vi "Initialize Single Node Browser.vi"(6 "Use Channel?":bool, 8 "error in (no error)":errorcluster, 9 "NodeName":string, 10 "Browser Ref 2":refnum<k24>, 11 "Item Ref in":T2 format="%.0x") -> (0 "error out":errorcluster, 2 "Browser Ref":T1, 3 "Item Ref out":T2 format="%.0x")   [LabVIEW 2015, in "Protection and Rolling Counter Addon System Explorer.lvlib"]
uses:
  <vilib>/NI Veristand/Custom Device API/Custom Device Item Ref.ctl
  NationalInstruments.VeriStand.SystemStorageUI
  <vilib>/NI Veristand/UI Controls/Single Node Browser/Single Node Browser Ref.ctl
  NationalInstruments.VeriStand.SystemStorage
  <vilib>/NI Veristand/Custom Device API/Get Item Property (Dependent Node Pointer).vi
  Protection and Rolling Counter Addon System Explorer.lvlib
  <vilib>/NI VeriStand/Custom Device Tools/Custom Device Utility Library/Custom Device Utility Library.lvlib
  <vilib>/NI VeriStand/Custom Device API/Custom Device API.lvlib
  <vilib>/NI Veristand/UI Controls/Single Node Browser/NI_VS UI Single Node Browser.lvlib
panel:
  in  "DisplayFilter":u8(ring)=7 items=["K_CHAN_R", "K_CHAN_W", "K_CHAN_RW", "K_CHAN_VOLT", "K_CHAN_FAULT", "K_ALL", "K_CUSTOM", "K_CHAN_R_VIS", "K_CHAN_W_VIS", "K_CHAN_RW_VIS", "K_CHAN_VOLT_VIS", "K_CHAN_FAULT_VIS"]
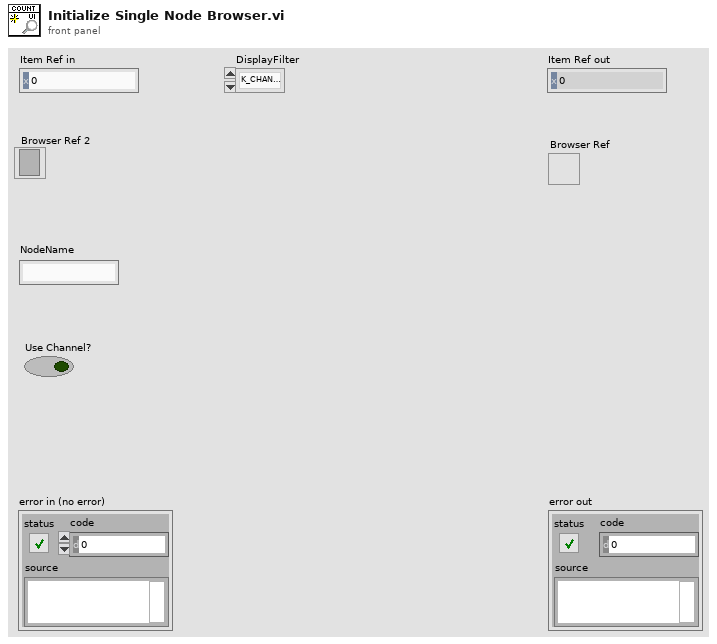
[diagram p1: front panel]
types:
  T1 = typedef "NI_VS UI Single Node Browser.lvlib/Single Node Browser Ref.ctl" = refnum<k24>
  T2 = typedef "Custom Device API.lvlib/Custom Device Item Ref.ctl" = u64
  T3 = typedef "Custom Device API.lvlib/Custom Device Pointer.ctl" = refnum<k24>
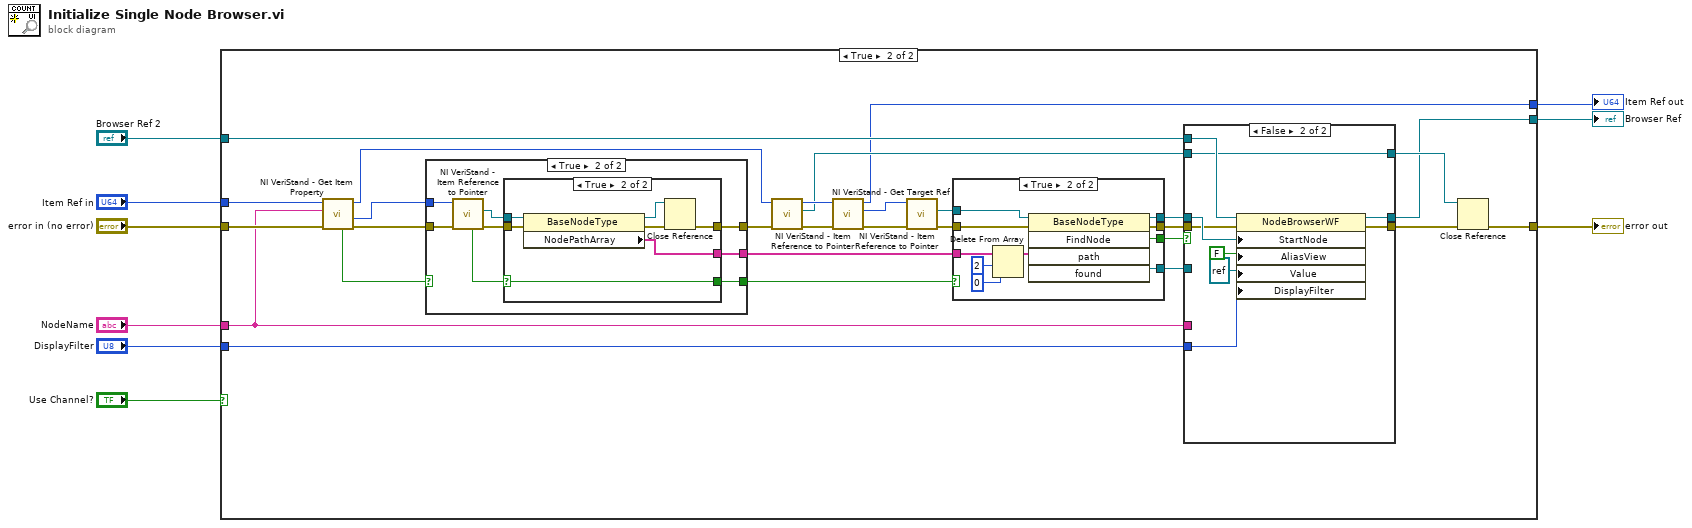
[diagram p0: block diagram]
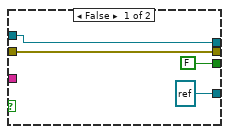
[diagram p5: hidden frame]
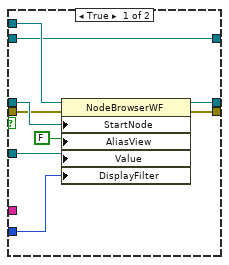
[diagram p6: hidden frame]
diagram:
  n1 = case shown="True" "Use Channel?" {
    tunnel: "DisplayFilter" -> [_ w39]
    tunnel: "Browser Ref 2" -> [w10 w31]
    tunnel: "Item Ref in" -> [w11 w29]
    tunnel: [w11 w26] -> w6
    tunnel: [w12 w24] -> w5
    tunnel: "error in (no error)" -> [w12 w22]
    tunnel: "NodeName" -> [_ w21]
    tunnel: [w10 w13] -> w2
    frame False {
    }
    frame True {
      n2 = call-poly <vilib>:"NI VeriStand - Get Item Property.vi"("error in (no error)"=w22, "Property Name"=w21, "Item Ref in"=w29) -> ("error out"=w19:errorcluster, "Dependent Node Ref"=w20:T2, "Item Ref out"=w23:T2, "Found"=w16:bool)  [unwired: 5 in]
      n3 = case shown="True" w16 {
        selector: w16 -> [w41 _]
        tunnel: w20 -> [_ w50]
        tunnel: w19 -> [w42 w49]
        tunnel: [w42 w46] -> w18
        tunnel: [_ w45] -> w15
        tunnel: [w41 w43] -> w17
        frame False {
        }
        frame True {
          n4 = call <vilib>:"NI VeriStand - Item Reference to Pointer.vi"("error in (no error)"=w49, "Item Ref in"=w50) -> ("error out"=w47:errorcluster, "Node Pointer"=w48:T3, "Found"=w44:bool)  [unwired: 6 in, 1 out]
          n5 = case shown="True" w44 {
            selector: w44 -> [w52 w56]
            tunnel: w48 -> [_ w59]
            tunnel: w47 -> [w51 w58]
            tunnel: [w51 w54] -> w46
            tunnel: [_ w57] -> w45
            tunnel: [w52 w56] -> w43
            frame False {
            }
            frame True {
              n6 = property class="BaseNodeType"(reference=w59, error in=w58) -> (reference out=w53:T3, error out=w55:errorcluster, "NodePathArray"=w57:string[])
              n7 = Close Reference(reference=w53, error in (no error)=w55) -> (error out=w54:errorcluster)
            }
          }
        }
      }
      n8 = call <vilib>:"NI VeriStand - Item Reference to Pointer.vi"("error in (no error)"=w18, "Item Ref in"=w23) -> ("error out"=w30:errorcluster, "Node Pointer"=w27:T3, "Item Ref out"=w28:T2)  [unwired: 6 in, 1 out]
      n9 = call <vilib>:"NI VeriStand - Get Target Ref.vi"("error in"=w30, "Item Ref in"=w28) -> ("error out"=w40:errorcluster, "Target Ref"=w33:T2, "Item Ref out"=w26:T2)  [unwired: 6 in, 1 out]
      n10 = call <vilib>:"NI VeriStand - Item Reference to Pointer.vi"("error in (no error)"=w40, "Item Ref in"=w33) -> ("error out"=w35:errorcluster, "Node Pointer"=w34:T3)  [unwired: 6 in, 2 out]
      n11 = case shown="True" w17 {
        tunnel: [refnum<k24> refnum ("Value") w73] -> w38
        tunnel: [w62 w72] -> w37
        tunnel: [w63 w71] -> w36
        tunnel: w35 -> [w63 w68]
        tunnel: w34 -> [w62 w70]
        tunnel: [FALSE ("FindNode") w69] -> w32
        tunnel: w15 -> [_ w65]
        frame False {
        }
        frame True {
          n12 = Delete From Array(array=w65, length=2, index=0) -> (array with subset deleted=w64:string[])  [unwired: 1 out]
          n13 = invoke class="BaseNodeType" method="FindNode"(reference=w70, error in=w68, "path"=w64) -> (reference out=w72:T3, error out=w71:errorcluster, "FindNode"=w69:bool, "found"=w73:refnum<k24>)  [unwired: 2 in, 1 out]
        }
      }
      n14 = case shown="False" w32 {
        tunnel: w39 -> [w78 w86]
        tunnel: w31 -> [w82 w91]
        tunnel: [w75 w83] -> w14
        tunnel: w37 -> [w81 w90]
        tunnel: w36 -> [w80 w89]
        tunnel: w38 -> [w79 _]
        tunnel: [w76 w88] -> w13
        tunnel: w27 -> [w74 w84]
        tunnel: [w74 w84] -> w25
        tunnel: w21 -> [_ _]
        frame True {
          n15 = property class="NodeBrowserWF"(reference=w82, error in=w80, "StartNode"=w81, "AliasView"=FALSE, "Value"=w79, "DisplayFilter"=w78) -> (reference out=w76:refnum<k24>, error out=w75:errorcluster)
        }
        frame False {
          n16 = property class="NodeBrowserWF"(reference=w91, error in=w89, "StartNode"=w90, "AliasView"=FALSE, "Value"=refnum<k24> refnum, "DisplayFilter"=w86) -> (reference out=w88:refnum<k24>, error out=w83:errorcluster)
        }
      }
      n17 = Close Reference(reference=w25, error in (no error)=w14) -> (error out=w24:errorcluster)
    }
  }
  "Item Ref out" <- w6
  "error out" <- w5
  "Browser Ref" <- w2
